vi "温度报警.vi"(0 "选择温度曲线":enum16{"温度1", "温度2", "温度3", "平均温度"}(ring)=enum."平均温度", 1 "温度曲线簇":T1, 3 "警示":refnum<vi>) -> (6 "预警":string)   [LabVIEW 2012]
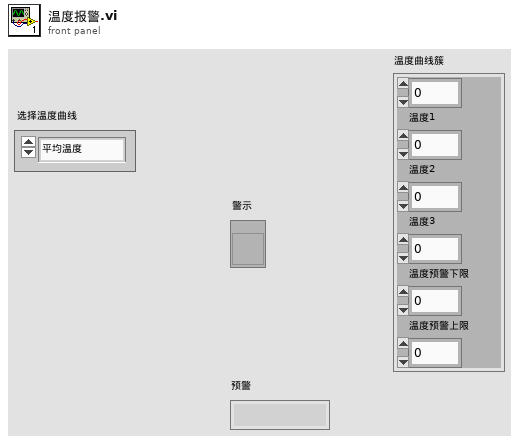
[diagram p1: front panel]
types:
  T1 = cluster{dbl, "温度1":dbl, "温度2":dbl, "温度3":dbl, "温度预警下限":dbl, "温度预警上限":dbl}
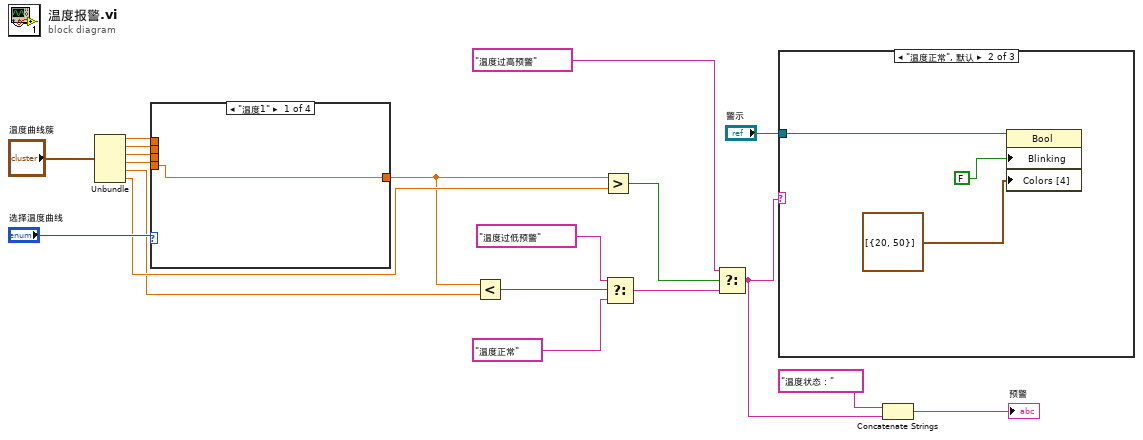
[diagram p0: block diagram]
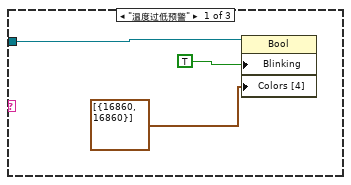
[diagram p5: hidden frame]
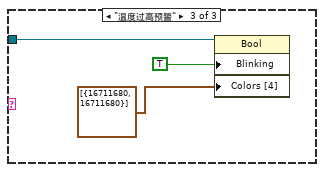
[diagram p6: hidden frame]
diagram:
  n1 = Unbundle("温度曲线簇") -> (w10:dbl, "温度1"=w9:dbl, "温度2"=w8:dbl, "温度3"=w7:dbl, "温度预警下限"=w5:dbl, "温度预警上限"=w6:dbl)
  n2 = case shown="\"温度1\"" "选择温度曲线" {
    tunnel: w10 -> [_ _ _ w23]
    tunnel: w9 -> [_ _ w22 _]
    tunnel: w8 -> [_ w21 _ _]
    tunnel: w7 -> [w20 _ _ _]
    tunnel: [w20 w21 w22 w23] -> w4
    frame "温度1" {
    }
    frame "温度2" {
    }
    frame "温度3" {
    }
    frame "平均温度", Default {
    }
  }
  n3 = Less?(x=w4, y=w5) -> (x < y?=w18:bool)
  n4 = Greater?(x=w4, y=w6) -> (0:w17:bool)
  n5 = Select(t="温度过低预警", s=w18, f="温度正常") -> (s? t:f=w14:string)
  n6 = Select(t="温度过高预警", s=w17, f=w14) -> (s? t:f=w2:string)
  n7 = case shown="\"温度正常\", 默认" w2 {
    tunnel: "警示" -> [w26 w29 w32]
    frame "温度过低预警" {
      n8 = property class="Bool"(reference=w26, "Blinking"=TRUE ("闪烁"), "Colors [4]"=cluster{u32, u32}[] [{16860, 16860}] ("颜色[4]")) -> ()  [unwired: 1 in, 2 out]
    }
    frame "温度正常", Default {
      n9 = property class="Bool"(reference=w29, "Blinking"=FALSE ("闪烁"), "Colors [4]"=cluster{u32, u32}[] [{20, 50}] ("颜色[4]")) -> ()  [unwired: 1 in, 2 out]
    }
    frame "温度过高预警" {
      n10 = property class="Bool"(reference=w32, "Blinking"=TRUE ("闪烁"), "Colors [4]"=cluster{u32, u32}[] [{16711680, 16711680}] ("颜色[4]")) -> ()  [unwired: 1 in, 2 out]
    }
  }
  n11 = Concatenate Strings("温度状态：" ("字符串"), w2) -> (→"预警":string)
